vi "8channel_RMS.vi"(7 "Apply":bool, 9 "sample length":i32=100, 11 "Input":dbl[](array[numeric])) -> (3 "RMS data array":dbl[](array[numeric]))   [LabVIEW 2023]
uses:
  <vilib>/ptbypt/NI_PtbyPt.lvlib
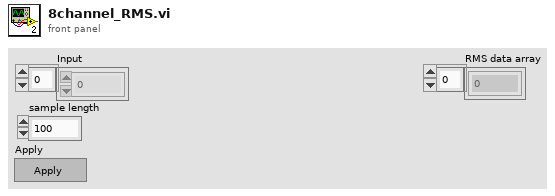
[diagram p1: front panel]
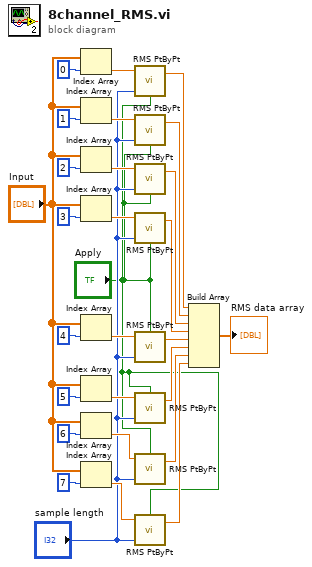
[diagram p0: block diagram]
diagram:
  n1 = Index Array(array="Input", index=0) -> (element=w19:dbl)
  n2 = Index Array(array="Input", index=1) -> (element=w18:dbl)
  n3 = Index Array(array="Input", index=2) -> (element=w17:dbl)
  n4 = Index Array(array="Input", index=3) -> (element=w16:dbl)
  n5 = Index Array(array="Input", index=4) -> (element=w15:dbl)
  n6 = Index Array(array="Input", index=5) -> (element=w14:dbl)
  n7 = Index Array(array="Input", index=6) -> (element=w13:dbl)
  n8 = Index Array(array="Input", index=7) -> (element=w12:dbl)
  n9 = call <vilib>:"RMS PtByPt.vi"("initialize"="Apply", "sample length"="sample length", "x"=w19) -> ("rms value"=w10:dbl)  [unwired: 1 in, 1 out]
  n10 = call <vilib>:"RMS PtByPt.vi"("initialize"="Apply", "sample length"="sample length", "x"=w18) -> ("rms value"=w9:dbl)  [unwired: 1 in, 1 out]
  n11 = call <vilib>:"RMS PtByPt.vi"("initialize"="Apply", "sample length"="sample length", "x"=w17) -> ("rms value"=w8:dbl)  [unwired: 1 in, 1 out]
  n12 = call <vilib>:"RMS PtByPt.vi"("initialize"="Apply", "sample length"="sample length", "x"=w16) -> ("rms value"=w7:dbl)  [unwired: 1 in, 1 out]
  n13 = call <vilib>:"RMS PtByPt.vi"("initialize"="Apply", "sample length"="sample length", "x"=w15) -> ("rms value"=w6:dbl)  [unwired: 1 in, 1 out]
  n14 = call <vilib>:"RMS PtByPt.vi"("initialize"="Apply", "sample length"="sample length", "x"=w14) -> ("rms value"=w5:dbl)  [unwired: 1 in, 1 out]
  n15 = call <vilib>:"RMS PtByPt.vi"("initialize"="Apply", "sample length"="sample length", "x"=w13) -> ("rms value"=w4:dbl)  [unwired: 1 in, 1 out]
  n16 = call <vilib>:"RMS PtByPt.vi"("initialize"="Apply", "sample length"="sample length", "x"=w12) -> ("rms value"=w3:dbl)  [unwired: 1 in, 1 out]
  n17 = Build Array(w10, w9, w8, w7, w6, w5, w4, w3) -> (→"RMS data array":dbl[])
